vi "set_new_position.vi"(8 "error in (no error)":errorcluster, 10 "set_pos":dbl[](array[numeric]), 11 "XPS in":refnum<class "XPS.lvclass">) -> (0 "error out":errorcluster, 3 "XPS out":refnum<class "XPS.lvclass">)   [LabVIEW 2019, in "XPS.lvlib" / "XPS.lvclass"]
uses:
  XPS.lvclass
  XPS.lvclass/XPS.ctl
  Newport.XPS.CommandInterface
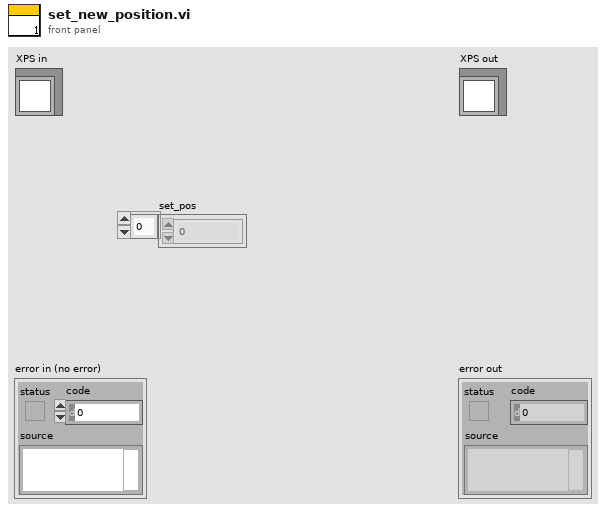
[diagram p1: front panel]
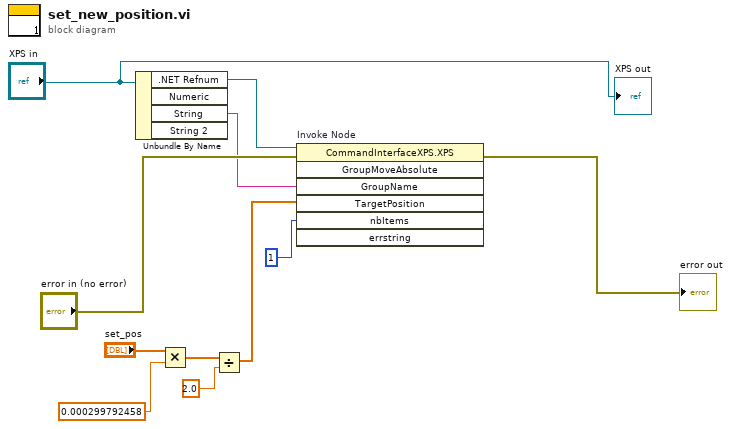
[diagram p0: block diagram]
diagram:
  n1 = Unbundle By Name("XPS in") -> (".NET Refnum"=w10:refnum<k24>, "String"=w1:string)  [unwired: 2 out]
  n2 = Multiply(x="set_pos", y=0.000299792458) -> (x*y=w6:dbl[])
  n3 = Divide(x=w6, y=2.0) -> (x/y=w2:dbl[])
  n4 = invoke on="Invoke Node" class="CommandInterfaceXPS.XPS" method="GroupMoveAbsolute"(reference=w10, error in="error in (no error)", "GroupName"=w1, "TargetPosition"=w2, "nbItems"=1) -> (error out=→"error out":errorcluster)  [unwired: 2 in, 6 out]
  "XPS out" <- "XPS in"
